vi "PI_GCS3_Configuration_Setup_ReferenceSwitch.vi"(0 "System no.":i32=1 min=1 step=1, 1 "Conn. Axes":string[](array[string]), 5 "error in":errorcluster) -> (14 "Has\nreference?":bool[](array[boolean]), 19 "error out":errorcluster)   [LabVIEW 2026]
doc: "Check which axes have a reference switch."
uses:
  SpecialCommand/ConfigurationMemoryType.ctl
panel:
  # "Check which axes have a reference switch."
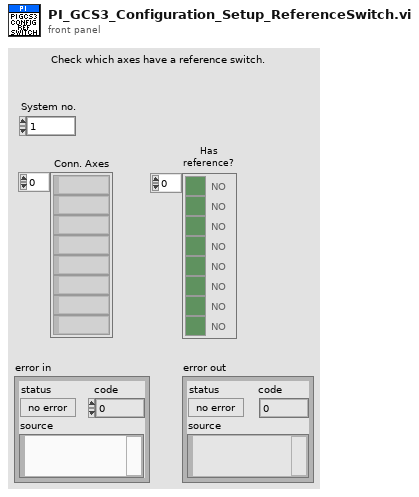
[diagram p1: front panel]
types:
  T1 = typedef "ConfigurationMemoryType.ctl" = enum16{"RAM", "TMP", "FLASH"}
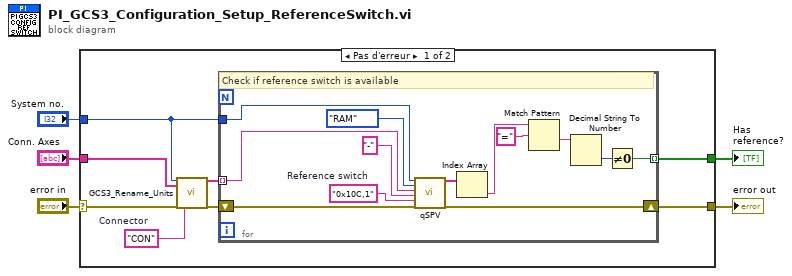
[diagram p0: block diagram]
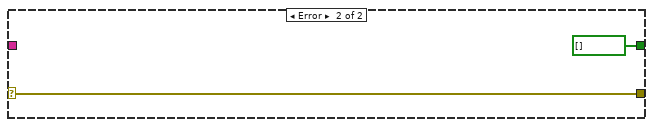
[diagram p2: hidden frame]
diagram:
  n1 = case shown="Pas d'erreur" "error in" {
    selector: "error in" -> [w11 w28]
    tunnel: [w13 w28] -> w2
    tunnel: "Conn. Axes" -> [w10 _]
    tunnel: "System no." -> [w9 _]
    tunnel: [w12 bool[] []] -> w1
    frame No Error {
      w6 = "CON"  # Connector
      n2 = call "GCS3_Rename_Units.vi"("System No."=w9, "Axes"=w10, "error in (no error)"=w11, "Target Unit"=w6) -> ("GCS 3.0 Units"=w8:string[], "error out"=w7:errorcluster)  [unwired: 14 in]
      n3 = for {
        shift-right: [w26] -> w13
        shift-left: w7 -> [w21]
        tunnel: w9 -> [w14]
        tunnel: w8 -> [w24] mode=indexing
        tunnel: [w15] -> w12 mode=indexing
        w25 = "0x10C,1"  # Reference switch
        # "Check if reference switch is available"
        n4 = call "qSPV.vi"("System no."=w14, "Target Memory Type"=ConfigurationMemoryType."RAM", "ContainerUnit"=w24, "FunctionUnit"="-", "ParameterID"=w25, "error in"=w21) -> ("Values"=w19:string[], "error out"=w26:errorcluster)  [unwired: 12 in]
        n5 = Index Array(array=w19) -> (element=w18:string)  [unwired: 1 in]
        n6 = Match Pattern(string=w18, regular expression="=") -> (after substring=w17:string)  [unwired: 1 in, 3 out]
        n7 = Decimal String To Number(string=w17) -> (number=w16:i32)  [unwired: 2 in, 1 out]
        n8 = Not Equal To 0?(x=w16) -> (x != 0?=w15:bool)
      }
    }
    frame Error {
    }
  }
  "error out" <- w2
  "Has\nreference?" <- w1
